vi "New Report Schema and Input Table Create.vi"(8 "error in":errorcluster, 11 "Schema":string="LTT_RESULT_INPUT_TABLES") -> (0 "error out":errorcluster)   [LabVIEW 2023]
uses:
  Database/SQL Public VI/Control/DB Options.ctl
  Database/Database.lvclass
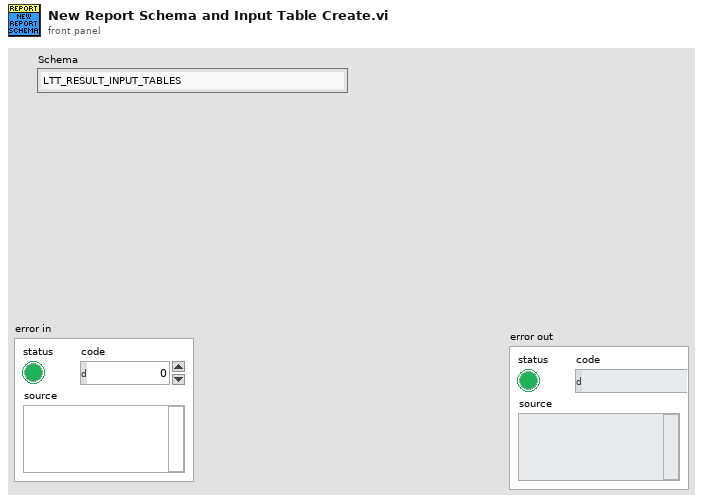
[diagram p1: front panel]
types:
  T1 = typedef "HardwareAbstractionLayer_LVOOP.lvlib/Database.lvclass/DB Options.ctl" = enum16{"Init", "Select Data", "Insert Data", "Update Data", "Delete Data", "Execute Query", "Create Schema", "Create Table", "List Tables", "List Columns", "Close"}
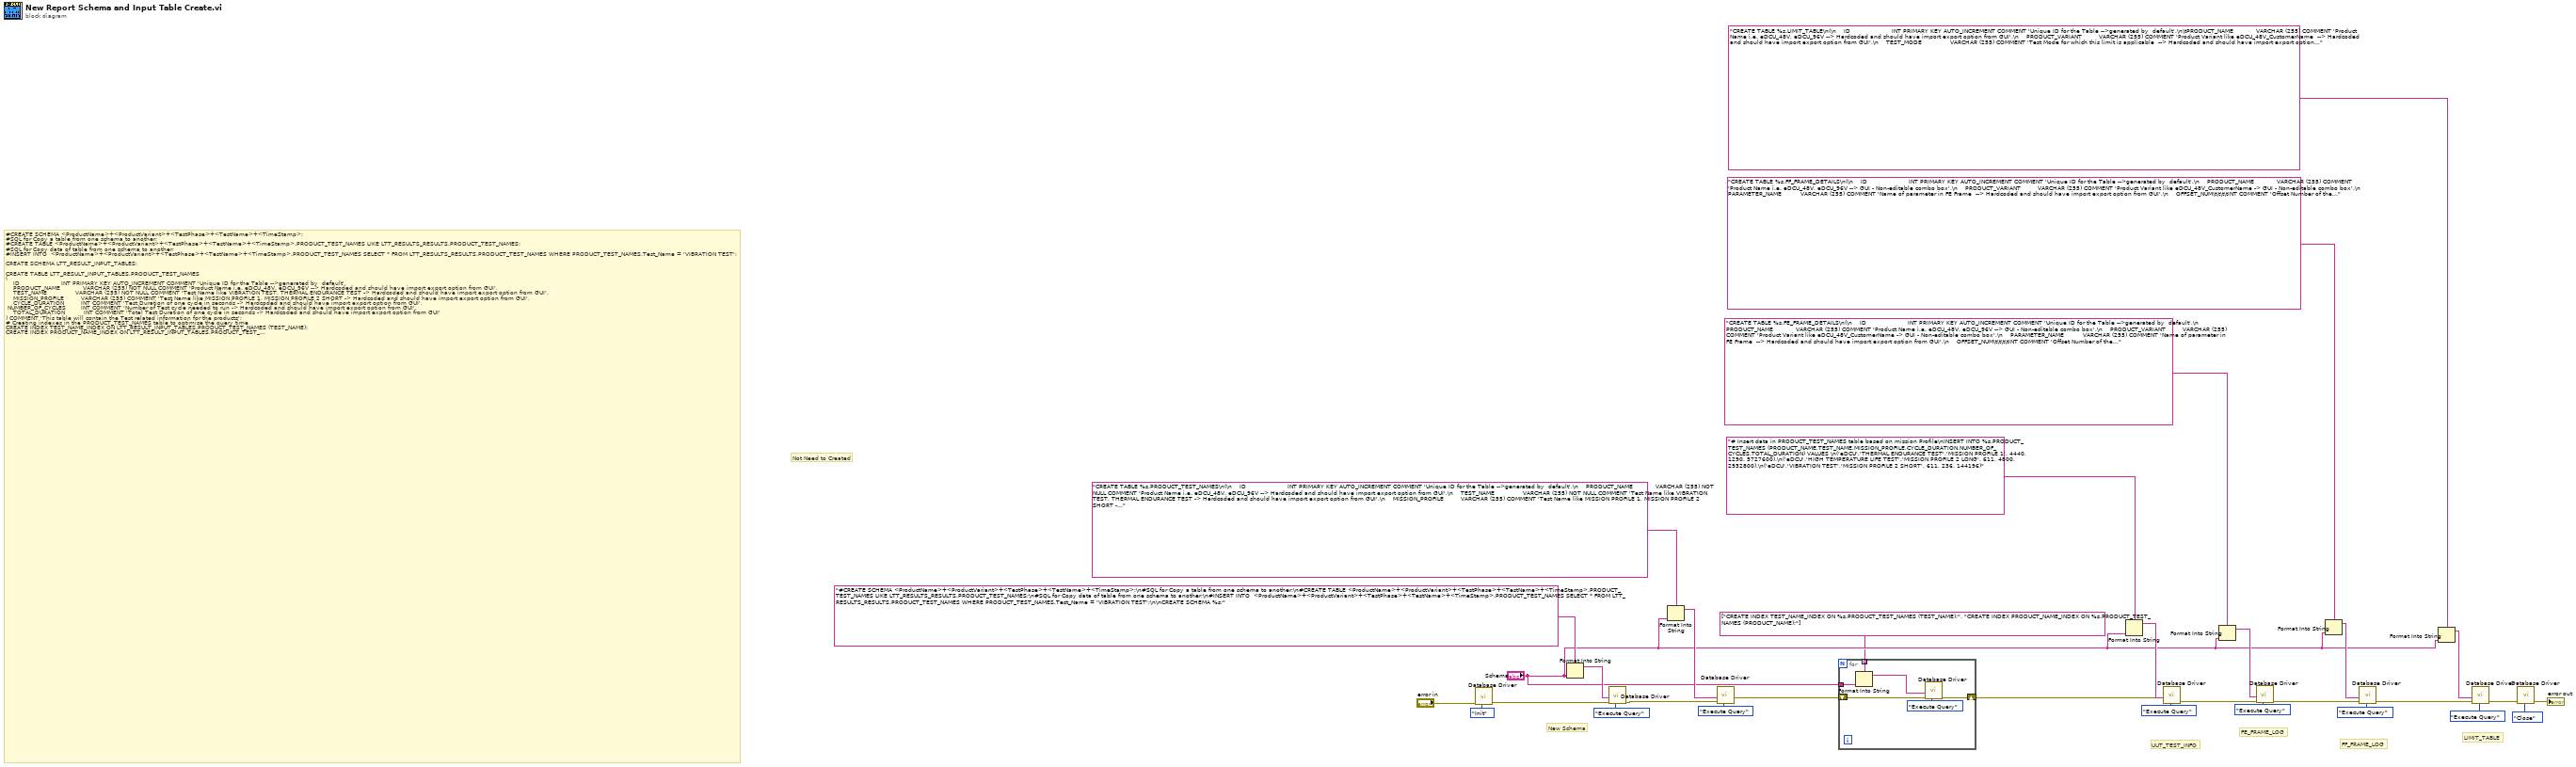
[diagram p0: block diagram]
diagram:
  # "Not Need to Created"
  # "#CREATE SCHEMA <ProductName>+<ProductVariant>+<TestPhase>+<TestName>+<TimeStamp>;\n#SQL for Copy a table from one schema to another;\n#CREATE TABLE <ProductName>+<ProductVariant>+<TestPhase>+<TestName>+<TimeStamp>.PRODUCT_TEST_NAMES LIKE LTT_RESULTS_RESULTS.PRODUCT_TEST_NAMES;\n#SQL for Copy data of table from one schema to another;\n#INSERT INTO  <ProductName>+<ProductVariant>+<TestPhase>+<TestName>+<TimeStamp>.PRODUCT_TEST_NAMES SELECT * FROM LTT_RESULTS_RESULTS.PRODUCT_TEST_NAMES WHERE PRODUCT_TEST_NAMES.Test_Name = 'VIBRATION TEST';\n\nCREATE SCHEMA LTT_RESULT_INPUT_TABLES;\n\nCREATE TABLE LTT_RESULT_INPUT_TABLES.PRODUCT_TEST_NAMES\n(\n    ID                      INT PRIMARY KEY AUTO_INCREMENT COMMENT 'Unique ID for the Table -->generated by  default',\n    PRODUCT_NAME            VARCHAR (255) NOT NULL COMMENT 'Product Name i.e. eDCU_48V, eDCU_96V --> Hardcoded and should have import export option from GUI',\n    TEST_NAME               VARCHAR (255) NOT NULL COMMENT 'Test Name like VIBRATION TEST, THERMAL ENDURANCE TEST -> Hardcoded and should have import export option from GUI',\n    MISSION_PROFILE         VARCHAR (255) COMMENT 'Test Name like MISSION PROFILE 1, MISSION PROFILE 2 SHORT -> Hardcoded and should have import export option from GUI',\n    CYCLE_DURATION\t        INT COMMENT 'Test Duration of one cycle in seconds -> Hardcoded and should have import export option from GUI',\n\tNUMBER_OF_CYCLES        INT COMMENT 'Number of Test cycle needed to run -> Hardcoded and should have import export option from GUI',\n    TOTAL_DURATION          INT\tCOMMENT 'Total Test Duration of one cycle in seconds -> Hardcoded and should have import export option from GUI'\n) COMMENT 'This table will contain the Test related information for the products';\n# Creating indexes in the PRODUCT_TEST_NAMES table to optimise the query time\nCREATE INDEX TEST_NAME_INDEX ON LTT_RESULT_INPUT_TABLES.PRODUCT_TEST_NAMES (TEST_NAME);\nCREATE INDEX PRODUCT_NAME_INDEX ON LTT_RESULT_INPUT_TABLES.PRODUCT_TEST_NAMES (PRODUCT_NAME);\n# Insert data in PRODUCT_TEST_NAMES table based on mission Profile\nINSERT INTO LTT_RESULT_INPUT_TABLES.PRODUCT_TEST_NAMES (PRODUCT_NAME,TEST_NAME,MISSION_PROFILE,CYCLE_DURATION,NUMBER_OF_CYCLES,TOTAL_DURATION) VALUES \n('eDCU','THERMAL ENDURANCE TEST','MISSION PROFILE 1', 4440, 1290, 5727600),\n('eDCU','HIGH TEMPERATURE LIFE TEST','MISSION PROFILE 2 LONG', 611, 4800, 2932800),\n('eDCU','VIBRATION TEST','MISSION PROFILE 2 SHORT', 611, 236, 144196)\n;\n\nCREATE TABLE LTT_RESULT_INPUT_TABLES.FE_FRAME_DETAILS\n(\n    ID                      INT PRIMARY KEY AUTO_INCREMENT COMMENT 'Unique ID for the Table -->generated by  default',\n    PRODUCT_NAME            VARCHAR (255) COMMENT 'Product Name i.e. eDCU_48V, eDCU_96V --> GUI - Non-editable combo box',\n    PRODUCT_VARIANT         VARCHAR (255) COMMENT 'Product Variant like eDCU_48V_CustomerName -> GUI - Non-editable combo box',\n    PARAMETER_NAME          VARCHAR (255) COMMENT 'Name of parameter in FE Frame  --> Hardcoded and should have import export option from GUI',\n    OFFSET_NUM\t\t\t\tINT COMMENT 'Offset Number of the Parameter in Return Data --> Hardcoded and should have import export option from GUI',\n    NB_BYTES\t\t\t\tINT\tCOMMENT 'Number of Bytes for the Parameter in Return Data --> Hardcoded and should have import export option from GUI',\n    CONVERSION_FORMULA      VARCHAR (255) COMMENT 'Conversion formula for the parameter ex. (x-32768)/16, optional --> Hardcoded and should have import export option from GUI'\n) COMMENT 'This table will store the details of FE Frames';\n\nCREATE TABLE LTT_RESULT_INPUT_TABLES.FF_FRAME_DETAILS\n(\n    ID                      INT PRIMARY KEY AUTO_INCREMENT COMMENT 'Unique ID for the Table -->generated by  default',\n    PRODUCT_NAME            VARCHAR (255) COMMENT 'Product Name i.e. eDCU_48V, eDCU_96V --> GUI - Non-editable combo box',\n    PRODUCT_VARIANT         VARCHAR (255) COMMENT 'Product Variant like eDCU_48V_CustomerName -> GUI - Non-editable combo box',\n    PARAMETER_NAME          VARCHAR (255) COMMENT 'Name of parameter in FE Frame  --> Hardcoded and should have import export option from GUI',\n    OFFSET_NUM\t\t\t\tINT COMMENT 'Offset Number of the Parameter in Return Data --> Hardcoded and should have import export option from GUI',\n    NB_BYTES\t\t\t\tINT\tCOMMENT 'Number of Bytes for the Parameter in Return Data --> Hardcoded and should have import export option from GUI',\n    CONVERSION_FORMULA      VARCHAR (255) COMMENT 'Conversion formula for the parameter ex. (x-32768)/16, optional --> Hardcoded and should have import export option from GUI'\n) COMMENT 'This table will store the details of FF Frames';\n\n\nCREATE TABLE LTT_RESULT_INPUT_TABLES.LIMIT_TABLE\n(\n    ID                      INT PRIMARY KEY AUTO_INCREMENT COMMENT 'Unique ID for the Table -->generated by  default',\n\tPRODUCT_NAME            VARCHAR (255) COMMENT 'Product Name i.e. eDCU_48V, eDCU_96V --> Hardcoded and should have import export option from GUI',\n    PRODUCT_VARIANT         VARCHAR (255) COMMENT 'Product Variant like eDCU_48V_CustomerName  --> Hardcoded and should have import export option from GUI',\n    TEST_MODE               VARCHAR (255) COMMENT 'Test Mode for which this limit is applicable  --> Hardcoded and should have import export option from GUI',\n    PARAMETER_NAME          VARCHAR (255) COMMENT 'Name of parameter for which this limit is applicable  --> Hardcoded and should have import export option from GUI',\n    COMPARISON_TYPE         VARCHAR (255) COMMENT 'Type of comparison like EQ(for EqualTo) OR GELE(for Greater than Equalto, Less than Equal to) --> Hardcoded and should have import export option from GUI',\n\tLOW_LIMIT               VARCHAR (255) COMMENT 'Low Limit for the Parameter OR Equal Value for the Parameter --> Hardcoded and should have import export option from GUI',\n    HIGH_LIMIT              VARCHAR (255) COMMENT 'Low Limit for the Parameter OR Equal Value for the Parameter --> Hardcoded and should have import export option from GUI',\n    UNIT                    VARCHAR (255) COMMENT 'Unit of  the Parameter --> Hardcoded and should have import export option from GUI',\n    ERROR_MESSSAGE          VARCHAR (255) COMMENT 'Error Message for the Parameter if it is out of range --> Hardcoded and should have import export option from GUI',\n    SEVERITY                VARCHAR (255) COMMENT 'Severity of the Parameter like NONE,CRITICAL, IGNORE, etc --> Hardcoded and should have import export option from GUI'\n) COMMENT 'This table will store the LIMIT data for FE/FF Frames';"
  # "LIMIT_TABLE"
  # "FF_FRAME_LOG"
  # "FE_FRAME_LOG"
  # "UUT_TEST_INFO"
  # "New Schema"
  n1 = call "Database Driver.vi"("Options"=DB_Options."Init", "error in"="error in") -> ("error out"=w30:errorcluster)  [unwired: 6 in, 3 out]
  n2 = Format Into String(format string="#CREATE SCHEMA <ProductName>+<ProductVariant>+<TestPhase>+<TestName>+<TimeStamp>;\n#SQL for Copy a table from one schema to another;\n#CREATE TABLE <ProductName>+<ProductVariant>+<TestPhase>+<TestName>+<TimeStamp>.PRODUCT_TEST_NAMES LIKE LTT_RESULTS_RESULTS.PRODUCT_TEST_NAMES;\n#SQL for Copy data of table from one schema to another;\n#INSERT INTO  <ProductName>+<ProductVariant>+<TestPhase>+<TestName>+<TimeStamp>.PRODUCT_TEST_NAMES SELECT * FROM LTT_RESULTS_RESULTS.PRODUCT_TEST_NAMES WHERE PRODUCT_TEST_NAMES.Test_Name = 'VIBRATION TEST';\n\nCREATE SCHEMA %s;", "Schema") -> (resulting string=w27:string)  [unwired: 2 in, 1 out]
  n3 = call "Database Driver.vi"("Options"=DB_Options."Execute Query", "error in"=w30, "SQL query"=w27) -> ("error out"=w7:errorcluster)  [unwired: 5 in, 3 out]
  n4 = Format Into String(format string="CREATE TABLE %s.PRODUCT_TEST_NAMES\n(\n    ID                      INT PRIMARY KEY AUTO_INCREMENT COMMENT 'Unique ID for the Table -->generated by  default',\n    PRODUCT_NAME            VARCHAR (255) NOT NULL COMMENT 'Product Name i.e. eDCU_48V, eDCU_96V --> Hardcoded and should have import export option from GUI',\n    TEST_NAME               VARCHAR (255) NOT NULL COMMENT 'Test Name like VIBRATION TEST, THERMAL ENDURANCE TEST -> Hardcoded and should have import export option from GUI',\n    MISSION_PROFILE         VARCHAR (255) COMMENT 'Test Name like MISSION PROFILE 1, MISSION PROFILE 2 SHORT -> Hardcoded and should have import export option from GUI',\n    CYCLE_DURATION\t        INT COMMENT 'Test Duration of one cycle in seconds -> Hardcoded and should have import export option from GUI',\n\tNUMBER_OF_CYCLES        INT COMMENT 'Number of Test cycle needed to run -> Hardcoded and should have import export option from GUI',\n    TOTAL_DURATION          INT\tCOMMENT 'Total Test Duration of one cycle in seconds -> Hardcoded and should have import export option from GUI'\n) COMMENT 'This table will contain the Test related information for the products';\n", "Schema") -> (resulting string=w6:string)  [unwired: 2 in, 1 out]
  n5 = call "Database Driver.vi"("Options"=DB_Options."Execute Query", "error in"=w7, "SQL query"=w6) -> ("error out"=w4:errorcluster)  [unwired: 5 in, 3 out]
  n6 = for {
    tunnel: "Schema" -> [w34]
    tunnel: string[] ["CREATE INDEX TEST_NAME_INDEX ON %s.PRODUCT_TEST_NAMES (TEST_NAME);", "CREATE INDEX PRODUCT_NAME_INDEX ON %s.PRODUCT_TEST_NAMES (PRODUCT_NAME);"] -> [w33] mode=indexing
    shift-right: [w37] -> w3
    shift-left: w4 -> [w38]
    n7 = Format Into String(format string=w33, w34) -> (resulting string=w36:string)  [unwired: 2 in, 1 out]
    n8 = call "Database Driver.vi"("Options"=DB_Options."Execute Query", "error in"=w38, "SQL query"=w36) -> ("error out"=w37:errorcluster)  [unwired: 5 in, 3 out]
  }
  n9 = Format Into String(format string="# Insert data in PRODUCT_TEST_NAMES table based on mission Profile\nINSERT INTO %s.PRODUCT_TEST_NAMES (PRODUCT_NAME,TEST_NAME,MISSION_PROFILE,CYCLE_DURATION,NUMBER_OF_CYCLES,TOTAL_DURATION) VALUES \n('eDCU','THERMAL ENDURANCE TEST','MISSION PROFILE 1', 4440, 1290, 5727600),\n('eDCU','HIGH TEMPERATURE LIFE TEST','MISSION PROFILE 2 LONG', 611, 4800, 2932800),\n('eDCU','VIBRATION TEST','MISSION PROFILE 2 SHORT', 611, 236, 144196)", "Schema") -> (resulting string=w15:string)  [unwired: 2 in, 1 out]
  n10 = call "Database Driver.vi"("Options"=DB_Options."Execute Query", "error in"=w3, "SQL query"=w15) -> ("error out"=w29:errorcluster)  [unwired: 5 in, 3 out]
  n11 = Format Into String(format string="CREATE TABLE %s.FE_FRAME_DETAILS\n(\n    ID                      INT PRIMARY KEY AUTO_INCREMENT COMMENT 'Unique ID for the Table -->generated by  default',\n    PRODUCT_NAME            VARCHAR (255) COMMENT 'Product Name i.e. eDCU_48V, eDCU_96V --> GUI - Non-editable combo box',\n    PRODUCT_VARIANT         VARCHAR (255) COMMENT 'Product Variant like eDCU_48V_CustomerName -> GUI - Non-editable combo box',\n    PARAMETER_NAME          VARCHAR (255) COMMENT 'Name of parameter in FE Frame  --> Hardcoded and should have import export option from GUI',\n    OFFSET_NUM\t\t\t\tINT COMMENT 'Offset Number of the Parameter in Return Data --> Hardcoded and should have import export option from GUI',\n    NB_BYTES\t\t\t\tINT\tCOMMENT 'Number of Bytes for the Parameter in Return Data --> Hardcoded and should have import export option from GUI',\n    CONVERSION_FORMULA      VARCHAR (255) COMMENT 'Conversion formula for the parameter ex. (x-32768)/16, optional --> Hardcoded and should have import export option from GUI'\n) COMMENT 'This table will store the details of FE Frames';\n" ("SQL query"), "Schema") -> (resulting string=w13:string)  [unwired: 2 in, 1 out]
  n12 = call "Database Driver.vi"("Options"=DB_Options."Execute Query", "error in"=w29, "SQL query"=w13) -> ("error out"=w22:errorcluster)  [unwired: 5 in, 3 out]
  n13 = Format Into String(format string="CREATE TABLE %s.FF_FRAME_DETAILS\n(\n    ID                      INT PRIMARY KEY AUTO_INCREMENT COMMENT 'Unique ID for the Table -->generated by  default',\n    PRODUCT_NAME            VARCHAR (255) COMMENT 'Product Name i.e. eDCU_48V, eDCU_96V --> GUI - Non-editable combo box',\n    PRODUCT_VARIANT         VARCHAR (255) COMMENT 'Product Variant like eDCU_48V_CustomerName -> GUI - Non-editable combo box',\n    PARAMETER_NAME          VARCHAR (255) COMMENT 'Name of parameter in FE Frame  --> Hardcoded and should have import export option from GUI',\n    OFFSET_NUM\t\t\t\tINT COMMENT 'Offset Number of the Parameter in Return Data --> Hardcoded and should have import export option from GUI',\n    NB_BYTES\t\t\t\tINT\tCOMMENT 'Number of Bytes for the Parameter in Return Data --> Hardcoded and should have import export option from GUI',\n    CONVERSION_FORMULA      VARCHAR (255) COMMENT 'Conversion formula for the parameter ex. (x-32768)/16, optional --> Hardcoded and should have import export option from GUI'\n) COMMENT 'This table will store the details of FF Frames';" ("SQL query"), "Schema") -> (resulting string=w11:string)  [unwired: 2 in, 1 out]
  n14 = call "Database Driver.vi"("Options"=DB_Options."Execute Query", "error in"=w22, "SQL query"=w11) -> ("error out"=w17:errorcluster)  [unwired: 5 in, 3 out]
  n15 = Format Into String(format string="CREATE TABLE %s.LIMIT_TABLE\n(\n    ID                      INT PRIMARY KEY AUTO_INCREMENT COMMENT 'Unique ID for the Table -->generated by  default',\n\tPRODUCT_NAME            VARCHAR (255) COMMENT 'Product Name i.e. eDCU_48V, eDCU_96V --> Hardcoded and should have import export option from GUI',\n    PRODUCT_VARIANT         VARCHAR (255) COMMENT 'Product Variant like eDCU_48V_CustomerName  --> Hardcoded and should have import export option from GUI',\n    TEST_MODE               VARCHAR (255) COMMENT 'Test Mode for which this limit is applicable  --> Hardcoded and should have import export option from GUI',\n    PARAMETER_NAME          VARCHAR (255) COMMENT 'Name of parameter for which this limit is applicable  --> Hardcoded and should have import export option from GUI',\n    COMPARISON_TYPE         VARCHAR (255) COMMENT 'Type of comparison like EQ(for EqualTo) OR GELE(for Greater than Equalto, Less than Equal to) --> Hardcoded and should have import export option from GUI',\n\tLOW_LIMIT               VARCHAR (255) COMMENT 'Low Limit for the Parameter OR Equal Value for the Parameter --> Hardcoded and should have import export option from GUI',\n    HIGH_LIMIT              VARCHAR (255) COMMENT 'Low Limit for the Parameter OR Equal Value for the Parameter --> Hardcoded and should have import export option from GUI',\n    UNIT                    VARCHAR (255) COMMENT 'Unit of  the Parameter --> Hardcoded and should have import export option from GUI',\n    ERROR_MESSSAGE          VARCHAR (255) COMMENT 'Error Message for the Parameter if it is out of range --> Hardcoded and should have import export option from GUI',\n    SEVERITY                VARCHAR (255) COMMENT 'Severity of the Parameter like NONE,CRITICAL, IGNORE, etc --> Hardcoded and should have import export option from GUI'\n) COMMENT 'This table will store the LIMIT data for FE/FF Frames';" ("SQL query"), "Schema") -> (resulting string=w9:string)  [unwired: 2 in, 1 out]
  n16 = call "Database Driver.vi"("Options"=DB_Options."Execute Query", "error in"=w17, "SQL query"=w9) -> ("error out"=w20:errorcluster)  [unwired: 5 in, 3 out]
  n17 = call "Database Driver.vi"("Options"=DB_Options."Close", "error in"=w20) -> ("error out"=→"error out":errorcluster)  [unwired: 6 in, 3 out]
